vi "PH_Sequencer.PC PPInternalTiming.vi"(0 "i ref in":refnum<vi>, 2 "Servicename":string, 3 "Waiting Time [s]":dbl=30.0, 4 "not linked?":bool, 5 "error in (no error)":errorcluster) -> (14 "i ref out":refnum<vi>, 19 "error out":errorcluster)   [LabVIEW 2014, in "PH_Sequencer.lvlib"]
doc: "This VI writes the remaining waiting time of the PU to own attributes."
uses:
  PH_Sequencer.lvlib
  PH_PowerUnit_BaseClass/PH_PowerUnit_BaseClass.PP PU Tags.ctl
  PH_PowerUnit_BaseClass/PH_PowerUnit_BaseClass.lvlib
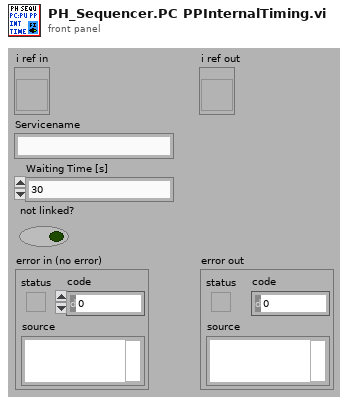
[diagram p1: front panel]
types:
  T1 = typedef "PH_Sequencer.lvlib/PH_Sequencer.i attribute.ctl" = cluster{"GUI Refs":cluster{"Main Off":refnum<vi>, "Fire":refnum<vi>, "Status":refnum<vi>, "Ready":refnum<vi>, "Waiting Time":refnum<vi>, "Timeout":refnum<vi>, "PPMA Ready":refnum<vi>, "Sequencer SM State":refnum<vi>, "PPPA Ready":refnum<vi>, "Calorimeter":refnum<vi>, "Beamline Ready":refnum<vi>, "Clear Beamline":refnum<vi>, "Linkage PPMA Rods":refnum<vi>, "Linkage Current PA":refnum<vi>, "Linkage Current MA":refnum<vi>, "Timing Ready":refnum<vi>, "State Timing":refnum<vi>, "Force Timing":refnum<vi>, "PSDB Shot Comment":refnum<vi>, "State PA Backreflection":refnum<vi>, "Beamline Z6 Ready":refnum<vi>, "Clear Z6 Beamline":refnum<vi>, "Sequence length":refnum<vi>, "Timing Mode":refnum<vi>, "Slow Trigger Settings":refnum<vi>, "Experiment Description":refnum<vi>, "State PSDB":refnum<vi>, "PSDB Ready":refnum<vi>, "Set PSDB Settings":refnum<vi>, "Get PSDB Info":refnum<vi>, "Take Snapshot":refnum<vi>, "Shottype":refnum<vi>, "Experiment":refnum<vi>, "Phase Frontends":refnum<vi>, "PP 45mm PILC in use":refnum<vi>}, "Status Info":cluster{"Machine Status":T2, "WaitingTime":i32, "Timeout":bool}, "Readyness":cluster{"Ready to shot":bool, "PPMA Ready":bool, "PPPA Ready":bool, "BL Ready":bool, "Timing Ready":bool, "BL Z6 Ready":bool, "PSDBReady":bool}, "Instancenames":cluster{"PPMA Rods":string, "PP Current Meas":string, "PH Beamline Chief":string, "PA Backrefl Meas":string, "Z6 Beamline Chief":string}, "Data to read":bool, "Calorimeter":cluster{"Instancename":string, "On":bool, "linked":bool}, "Linkage":cluster{"PPMA Rods":bool, "PP Current Meas":bool, "PHELIX Beamline Chief":bool, "PA Backrefl Meas":bool, "Z6 Beamline Chief":bool}, "Timing":cluster{"Instance":string, "linked":bool, "Status":T2, "Timing Mode":T3, "Slow Trigger Settings":T4, "Info available":cluster{"ext SlowTrigger":bool, "T2":bool, "Mode":bool, "Delay Slow Trigger":bool, "Phase FEs":bool}, "FE Phase":T5}, "Service ID R2S":i32, "PSDB":cluster{"Controller Instance":string, "Controller Status":T2, "Controller linked":bool, "Settings acknowledged":bool, "Current Experiment ID":i16, "Current Shot Type":i16, "Current Comment":string, "Remember Settings":bool, "Write 2 early":bool}, "PSDB Data":cluster{"Main Off?":bool, "Sequence Length":dbl, "Sequence startet":timestamp}, "6P 4Q Positions":cluster{"Instancename":string, "linked":bool, "Position":T6}[], "PUs":T7[]}
  T2 = typedef "PH_StatusHandler.lvlib/PH_StatusHandler.Status.ctl" = i16
  T3 = typedef "PH_Timing.lvlib/PH_Timing.Timing Mode.ctl" = cluster{"T2":i16, "Modeselector":enum32{"10 Hz", "0.5 Hz", "Shot"}}
  T4 = typedef "PH_Timing.lvlib/PH_Timing.Slow Trigger Settings.ctl" = cluster{"Delay":dbl, "externally triggered?":bool}
  T5 = typedef "PH_Timing.lvlib/PH_Timing.Phase FEs.ctl" = cluster{"Phase":dbl}
  T6 = typedef "PH_4_Pos_Selector.lvlib/PH_4_Pos_Selector.Position Selector.ctl" = u16
  T7 = typedef "PH_Sequencer.lvlib/PH_Sequencer.Head.ctl" = cluster{"PowerUnit":T8, "GUI Ref":refnum<vi>, "Information":T9, "linked?":bool, "GUI Ref Current Voltage":refnum<vi>}
  T8 = typedef "PH_PP_Common.lvlib/PH_PP_Common.PUs.ctl" = enum16{"no Info", "PA-19mm-1", "PA-19mm-2", "PA-45mm-PILC", "PA-45mm-MAIN", "MA-PU-1", "MA-PU-2", "MA-PU-3", "MA-PU-4", "MA-PU-5", "MA-PU-6", "MA-FR", "MA-PILC", "PA-45mm-DP"}
  T9 = typedef "PH_Sequencer.lvlib/PH_Sequencer.PU Information.ctl" = cluster{"State":T2, "Waiting Time [s]":dbl, "PU State SM":T10, "PU Timeout SM":T10}
  T10 = typedef "PH_PowerUnit_BaseClass.lvlib/PH_PowerUnit_BaseClass.SM States.ctl" = enum16{".", "Stand by", "Switch PU on", "Configure", "Set Default Voltage", "Set STANDBY", "Set READY", "Wait for Shot Cmd", "Open Dump Rods", "Open Ross Relais", "Close Ross Relais", "Switch PSU on", "Switch PSU off", "Charge", "Switch GD Channel on", "Close Dump Rods", "Rods-TO", "RR-TO", "PSU-TO", "Trigger-TO"}
  T11 = typedef "PH_PowerUnit_BaseClass.lvlib/PH_PowerUnit_BaseClass.PP PU Tags.ctl" = enum16{"Waiting-Time", "PU-in-Use"}
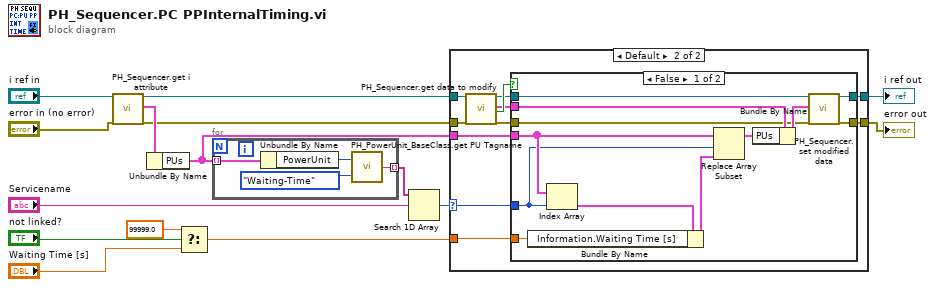
[diagram p0: block diagram]
diagram:
  n1 = call "PH_Sequencer.get i attribute.vi"("i ref in"="i ref in", "error in (no error)"="error in (no error)") -> ("i ref out"=w2:refnum<vi>, "i attribute"=w9:T1, "error out"=w1:errorcluster)  [unwired: 15 in]
  n2 = Unbundle By Name(w9) -> ("PUs"=w6:T7[])
  n3 = Select(t=99999.0, s="not linked?", f="Waiting Time [s]") -> (s? t:f=w12:dbl)
  n4 = for {
    tunnel: w6 -> [w19] mode=indexing
    tunnel: [w16] -> w7 mode=indexing
    n5 = Unbundle By Name(w19) -> ("PowerUnit"=w18:T8)
    n6 = call "PH_PowerUnit_BaseClass.get PU Tagname.vi"("PU Tag"=PH_PowerUnit_BaseClass.PP_PU_Tags."Waiting-Time", "PU"=w18) -> ("PU Tagname"=w16:string)
  }
  n7 = Search 1D Array(1D array=w7, element="Servicename") -> (index of element=w5:i32)  [unwired: 1 in]
  n8 = case shown="Default" w5 {
    selector: w5 -> [_ w23]
    tunnel: w12 -> [_ w31]
    tunnel: [w20 w29] -> w14
    tunnel: [w21 w27] -> w15
    tunnel: w1 -> [w20 w25]
    tunnel: w2 -> [w21 w24]
    tunnel: w6 -> [_ w22]
    frame -1 {
    }
    frame Default {
      n9 = call "PH_Sequencer.get data to modify.vi"("i ref in"=w24, "error in (no error)"=w25) -> ("i ref out"=w26:refnum<vi>, "i attribute"=w30:T1, "timed out"=w32:bool, "error out"=w28:errorcluster)  [unwired: 14 in]
      n10 = case shown="False" w32 {
        tunnel: w26 -> [w44 w46]
        tunnel: [w43 w46] -> w27
        tunnel: w28 -> [w39 w45]
        tunnel: [w42 w45] -> w29
        tunnel: w30 -> [w40 _]
        tunnel: w31 -> [w38 _]
        tunnel: w23 -> [w34 _]
        tunnel: w22 -> [w36 _]
        frame False {
          n11 = Index Array(array=w36, index=w34) -> (element=w37:T7)
          n12 = Bundle By Name(cluster=w37, "Information.Waiting Time [s]"=w38) -> (w35:T7)
          n13 = Replace Array Subset(array=w36, new element=w35, index=w34) -> (w33:T7[])
          n14 = Bundle By Name(cluster=w40, "PUs"=w33) -> (w41:T1)
          n15 = call "PH_Sequencer.set modified data.vi"("i ref in"=w44, "i attribute"=w41, "error in (no error)"=w39) -> ("i ref out"=w43:refnum<vi>, "error out"=w42:errorcluster)  [unwired: 15 in]
        }
        frame True {
        }
      }
    }
  }
  "error out" <- w14
  "i ref out" <- w15
